vi "CleanUp.vi"(8 "Error In":errorcluster, 11 "Object in":refnum<class "2021_01.lvclass">) -> (0 "Error Out":errorcluster, 3 "object out":refnum<class "2021_01.lvclass">)   [LabVIEW 2020]
uses:
  2021_01.lvclass/2021_01.ctl
  2021_01.lvclass
  C:/Projects/AdventCode/PuzzleBase_class/PuzzleBase.lvclass
  C:/Projects/AdventCode/PuzzleClasses/2021_01_class/2021_01.lvclass
  <resource>/Framework/Providers/Open_GDS/ClassProviders/Provider_LvNativeClass/Templates/NativeSubTemplate_4x4x4/NativeSubTemplate_4x4x4.lvclass
  C:/Program Files/National Instruments/LabVIEW 2020/resource/Framework/Providers/Open_GDS/ClassProviders/Provider_LvNativeClass/Templates/NativeBaseTemplate_4x4x4/NativeBaseTemplate_4x4x4.lvclass
  C:/Program Files/National Instruments/LabVIEW 2020/resource/Framework/Providers/Open_GDS/ClassProviders/Provider_LvNativeClass/Templates/NativeSubTemplate_4x4x4/NativeSubTemplate_4x4x4.lvclass
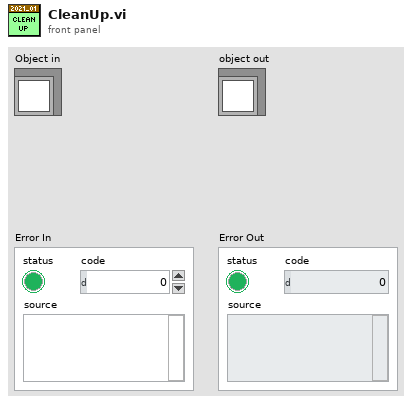
[diagram p1: front panel]
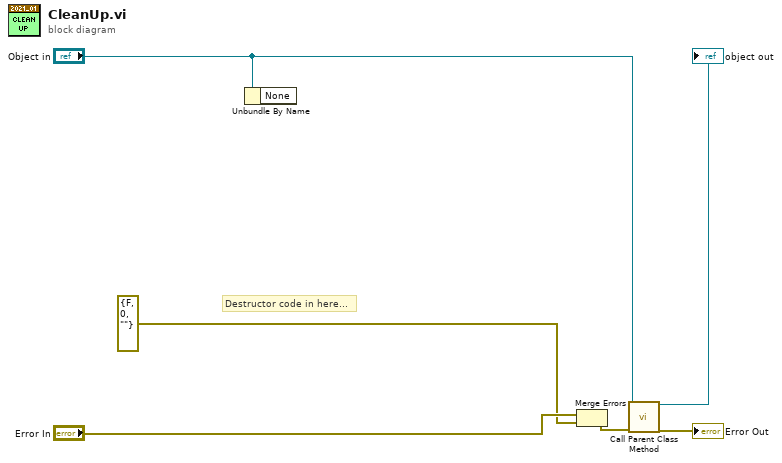
[diagram p0: block diagram]
diagram:
  # "Destructor code in here..."
  n1 = Unbundle By Name("Object in") -> ()  [unwired: 1 out]
  n2 = Merge Errors("Error In", errorcluster {"status"=FALSE, "code"=0, "source"=""} ("error in (no error)")) -> (w2:errorcluster)
  n3 = call-parent "Call Parent Class Method"("Error In"=w2, "object in"="Object in") -> ("Error Out"=→"Error Out":errorcluster, "object out"=→"object out":refnum<class "NativeSubTemplate_4x4x4.lvclass">)  [unwired: 8 in]
